vi "NT Get Persistence.vi"(8 "error in":errorcluster, 11 "Name":string="Numeric") -> (0 "error out":errorcluster, 3 "Persistence":bool=TRUE)   [LabVIEW 2020]
doc: "Read whether the topic is persistent ... will it be saved and loaded back next time the program boots up?"
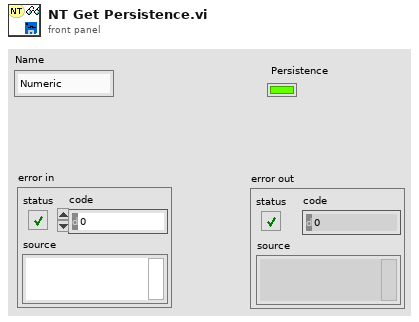
[diagram p1: front panel]
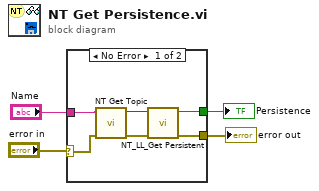
[diagram p0: block diagram]
diagram:
  n1 = case shown="No Error" "error in" {
    selector: "error in" -> [w9 w11]
    tunnel: "Name" -> [w10 _]
    tunnel: [w5 w11] -> w2
    tunnel: [w6 _] -> w1
    frame No Error {
      n2 = call "NT Get Topic.vi"("error in (no error)"=w9, "name"=w10) -> ("error out"=w7:errorcluster, "topicHandle"=w8:u32)  [unwired: 8 in]
      n3 = call "NT_LL_Get Persistent.vi"("error in (no error)"=w7, "topicHandle"=w8) -> ("error out"=w5:errorcluster, "Boolean"=w6:bool)  [unwired: 8 in]
    }
    frame Error {
    }
  }
  "error out" <- w2
  "Persistence" <- w1
